vi "SplashWnd - Module Starting Up2.vi"(4 "LoadingWait(ms)":u32=100, 5 "VI Ref (calling VI)":refnum<vi>, 6 "Prototypes":refnum<vi>[](array[refnum]), 7 "Title":string, 8 "error in (no error)":errorcluster, 9 "Name (\"\" to Use UUID)":string="SplashWindow", 11 "Array":cluster{"ModuleName":string, "Index":i32}[](array[cluster])) -> (0 "error out":errorcluster)   [LabVIEW 2020, in "CSM-SplashWindow.lvlib"]
uses:
  CSM-SplashWindow.lvlib
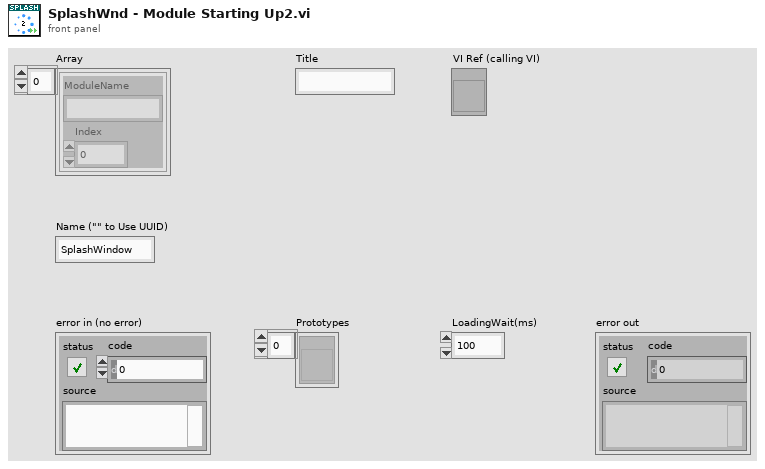
[diagram p1: front panel]
types:
  T1 = enum32{"Invalid", "Standard", "Closed", "Hidden", "Minimized", "Maximized"}
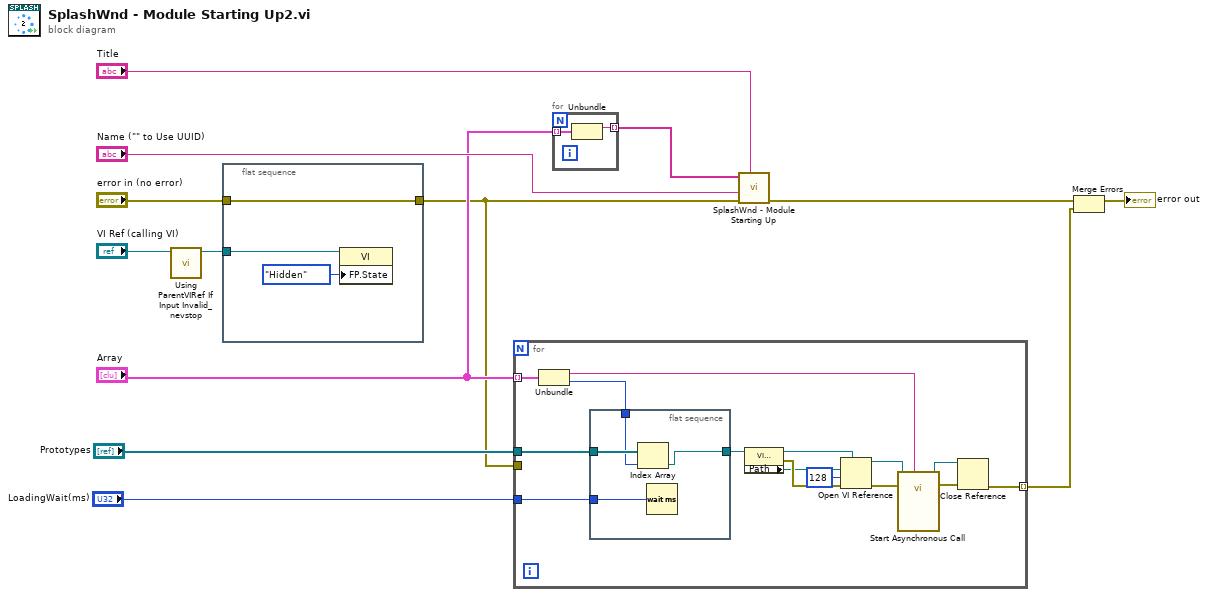
[diagram p0: block diagram]
diagram:
  n1 = call <userlib>:"Using ParentVIRef If Input Invalid_nevstop.vi"("VI Ref (calling VI)"="VI Ref (calling VI)") -> ("VI Ref"=w3:refnum<vi>)  [unwired: 5 in, 1 out]
  n2 = flat-sequence {
    tunnel: w3 -> [w16]
    tunnel: "error in (no error)" -> [w14]
    tunnel: [w14] -> w1
    frame #0 {
      n3 = property class="VI"(reference=w16, "FP.State"=T1."Hidden" ("Front Panel Window:State")) -> ()  [unwired: 1 in, 2 out]
    }
  }
  n4 = for {
    tunnel: "Array" -> [w25] mode=indexing
    tunnel: "Prototypes" -> [w24]
    tunnel: [w20] -> w12 mode=indexing
    tunnel: w1 -> [_]
    tunnel: "LoadingWait(ms)" -> [w17]
    n5 = Unbundle(w25) -> ("ModuleName"=w23:string, "Index"=w21:i32)
    n6 = flat-sequence {
      tunnel: w24 -> [w35]
      tunnel: [w34] -> w22
      tunnel: w21 -> [w33]
      tunnel: w17 -> [w32]
      frame #0 {
        n7 = Index Array(array=w35, index=w33) -> (element=w34:refnum<vi>)
        n8 = Wait (ms)(milliseconds to wait=w32) -> ()  [unwired: 1 out]
      }
    }
    n9 = property class="VI (strict)"(reference=w22) -> (reference out=w28:refnum<vi>, error out=w27:errorcluster, "Path"=w26:path)  [unwired: 1 in]
    n10 = Open VI Reference(type specifier VI Refnum (for type only)=w28, vi path=w26, options=128, error in (no error)=w27) -> (vi reference=w18:refnum<vi>, error out=w19:errorcluster)  [unwired: 2 in]
    n11 = call-by-ref "Start Asynchronous Call"(reference=w18, error in=w19, "Name (\"\" to Use UUID)"=w23) -> (reference out=w30:refnum<vi>, error out=w29:errorcluster)  [unwired: 11 in]
    n12 = Close Reference(reference=w30, error in (no error)=w29) -> (error out=w20:errorcluster)
  }
  n13 = for {
    tunnel: "Array" -> [w37] mode=indexing
    tunnel: [w36] -> w8 mode=indexing
    n14 = Unbundle(w37) -> ("ModuleName"=w36:string)  [unwired: 1 out]
  }
  n15 = call "SplashWnd - Module Starting Up.vi"("Title"="Title", "Error In (No Error)"=w1, "Name (\"\" to Use UUID)"="Name (\"\" to Use UUID)", "Modules"=w8) -> ("error out"=w10:errorcluster)  [unwired: 7 in]
  n16 = Merge Errors(w10, w12) -> (→"error out":errorcluster)
